vi "Main_011.vi"() -> ()   [LabVIEW 2025]
uses:
  Utility/Universal Utility/TypeDefs_Utility/ENUM_8 Directions U-D-L-R.ctl
  9e3f57c0-2ef8-4495-8287-c6a42a5fb955.vi
  <vilib>/Utility/error.llb/Trim Whitespace.vi
  <vilib>/Utility/error.llb/Trim Whitespace One-Sided.vi
  Utility/Universal Utility/TypeDefs_Utility/Cluster_Row-Column.ctl
  Utility/Universal Utility/TypeDefs_Utility/ENUM_4 Directions U-D-L-R.ctl
panel:
  out "Array":i32[][](array[numeric])
  in  "Puzzle Input":u64=4
  in  "Puzzle Target":u64=70600674
  in  "Data":string
  out "MATCH":bool
  out "Answer":u64
  # "MAX Product in Grid"
  # "Number of same direction numbers\n(Up, Down, Left, Right  Diaganal)"
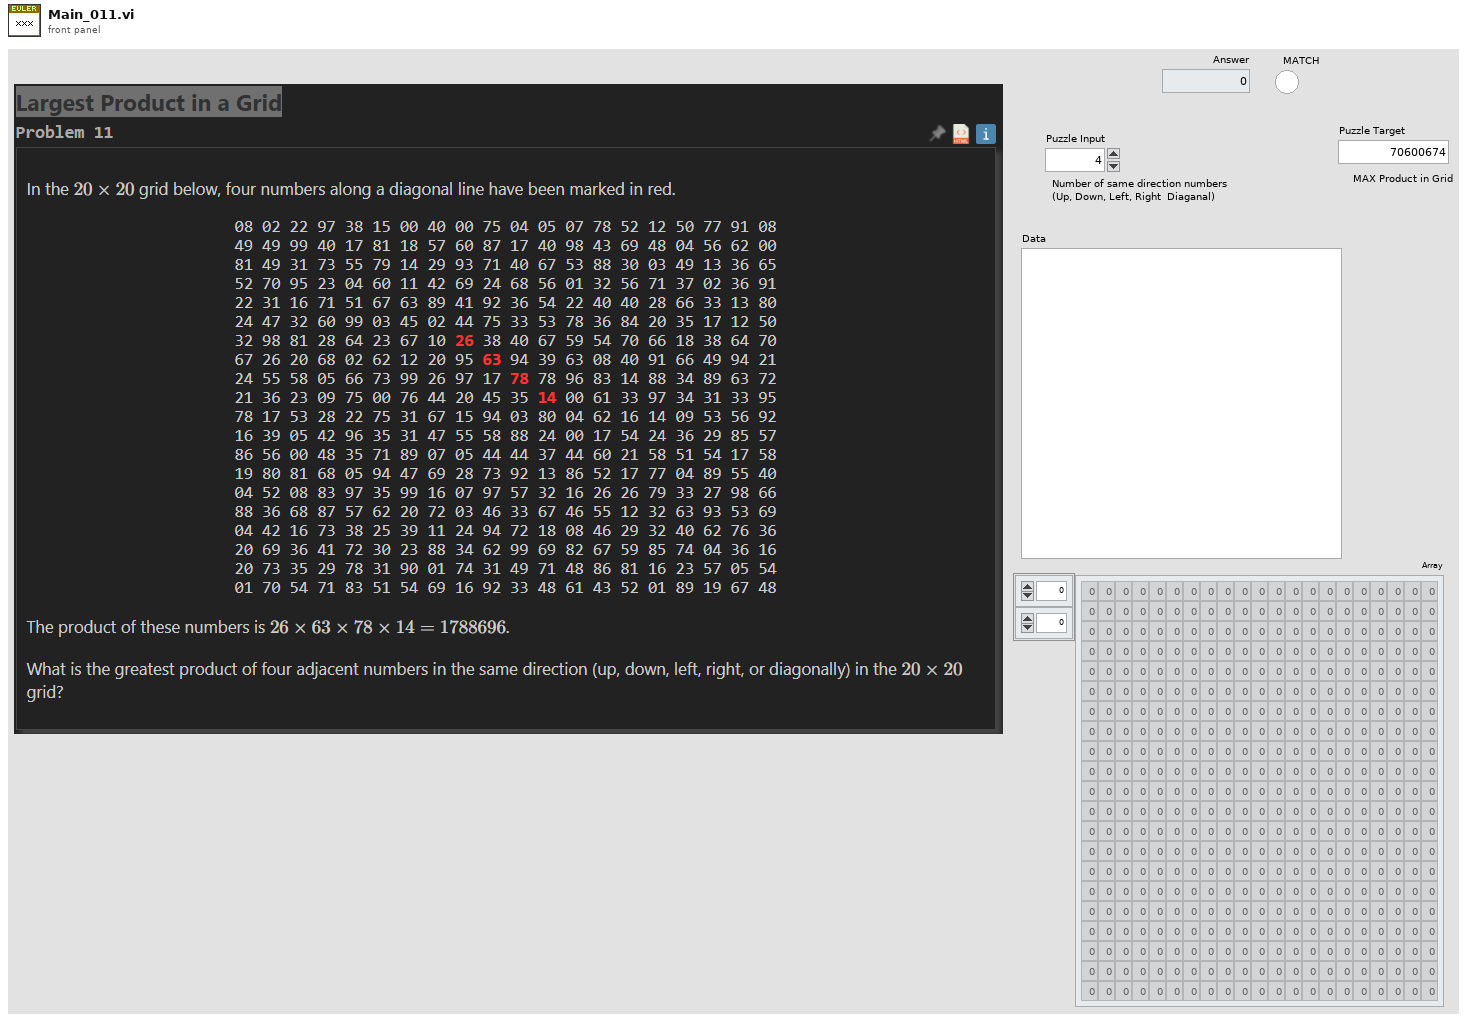
[diagram p1: front panel]
types:
  T1 = typedef "ENUM_4 Directions U-D-L-R.ctl" = enum16{"Up;-1,0", "Right;0,1", "Down;1,0", "Left;0,-1"}
  T2 = typedef "Cluster_Row-Column.ctl" = cluster{"R":i32, "C":i32}
  T3 = typedef "ENUM_8 Directions U-D-L-R.ctl" = enum16{"Up;-1,0", "Up-Right;-1,1", "Right;0,1", "Down-Right;1,1", "Down;1,0", "Down-Left;1,-1", "Left;0,-1", "Up-Left;-1,-1"}
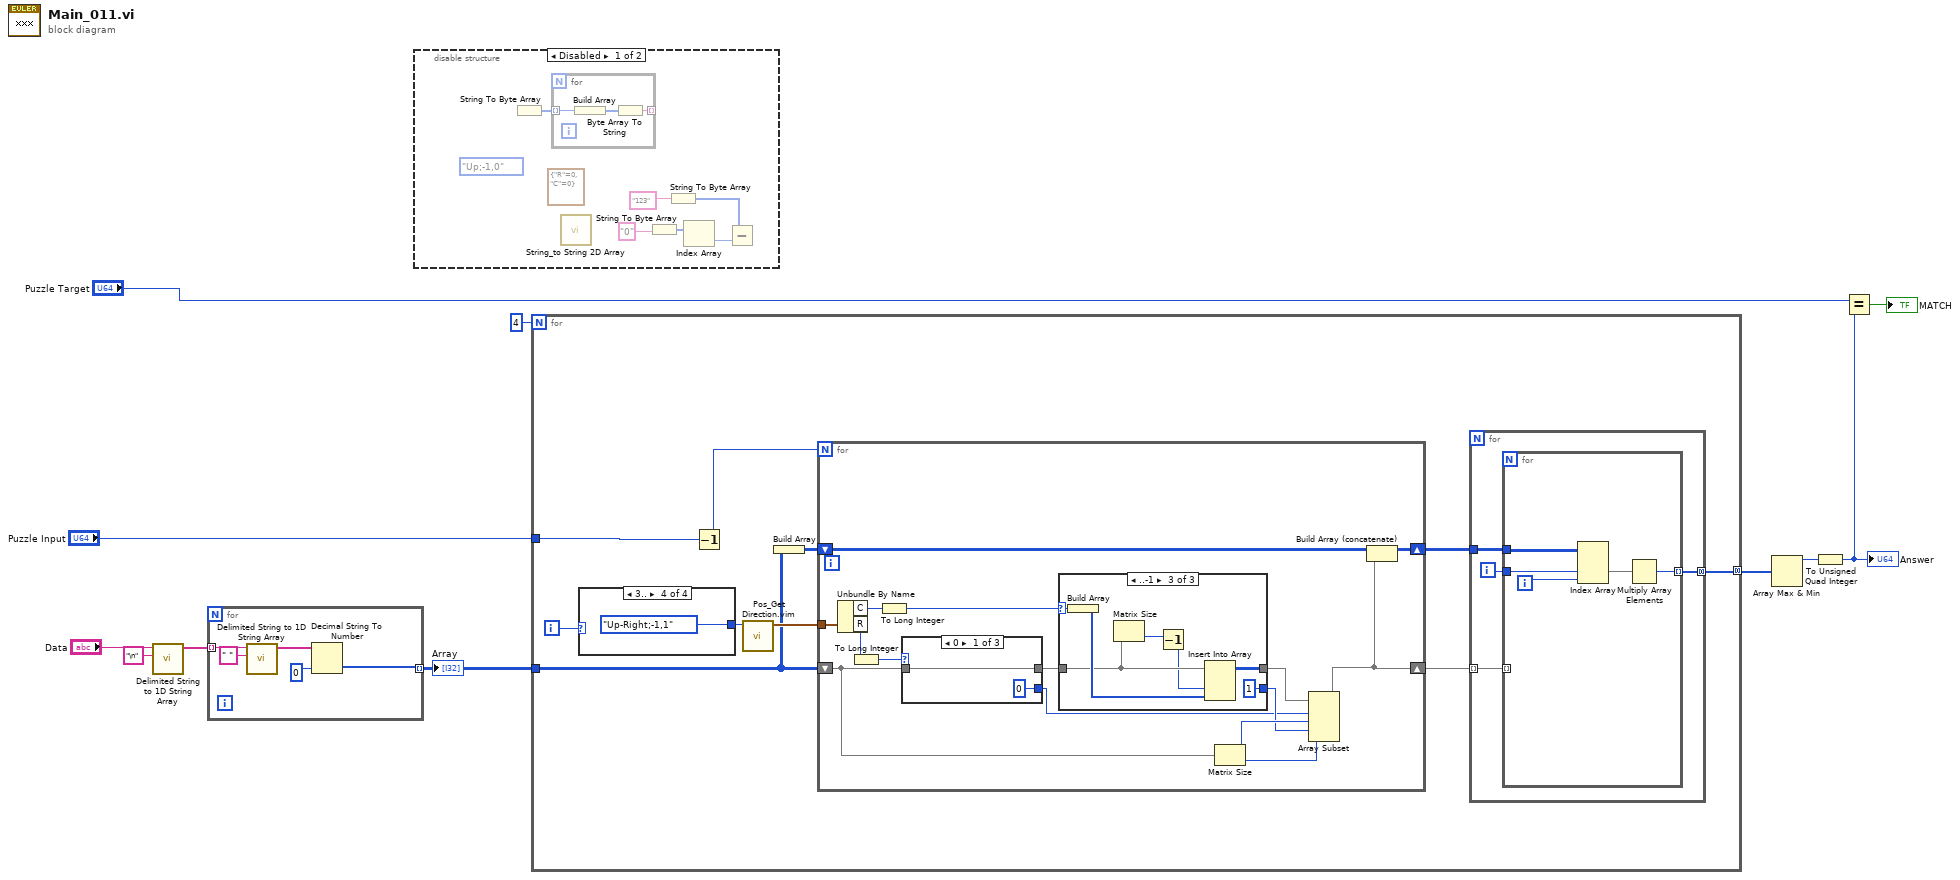
[diagram p0: block diagram]
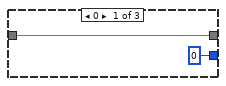
[diagram p2: hidden frame]
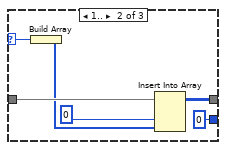
[diagram p3: hidden frame]
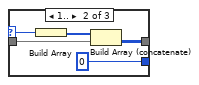
[diagram p4: hidden frame]
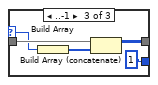
[diagram p5: hidden frame]
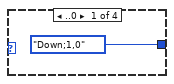
[diagram p6: hidden frame]
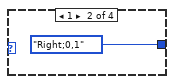
[diagram p7: hidden frame]
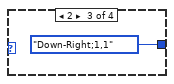
[diagram p8: hidden frame]
diagram:
  n1 = call <vilib>:"Delimited String to 1D String Array.vi"("delimiter"="\n", "delimited string"="Data") -> ("string array"=w6:string[])  [unwired: 9 in]
  n2 = for {
    tunnel: w6 -> [w16] mode=indexing
    tunnel: [w12] -> w4 mode=indexing
    n3 = call <vilib>:"Delimited String to 1D String Array.vi"("delimiter"=" ", "delimited string"=w16) -> ("string array"=w13:string[])  [unwired: 9 in]
    n4 = Decimal String To Number(string=w13, default (0L)=0 ("default (0 I32)")) -> (number=w12:i32[])  [unwired: 1 in, 1 out]
  }
  "Array" <- w4
  n5 = disable-structure shown="Disabled" {
    frame Disabled {
      (unwired) ENUM_4_Directions_U-D-L-R."Up;-1,0" ("Direction")
      (unwired) T2 {"R"=0, "C"=0} ("Position")
      n6 = String To Byte Array() -> (unsigned byte array=w17:u8[])  [unwired: 1 in]
      n7 = for {
        tunnel: w17 -> [w25] mode=indexing
        tunnel: [w23] -> _ mode=indexing
        n8 = Build Array(w25) -> (w24:u8[])
        n9 = Byte Array To String(unsigned byte array=w24) -> (string=w23:string)
      }
      n10 = call "String_to String 2D Array.vi"() -> ()  [unwired: 11 in, 1 out]
      n11 = String To Byte Array(string="0") -> (unsigned byte array=w20:u8[])
      n12 = String To Byte Array(string="123") -> (unsigned byte array=w18:u8[])
      n13 = Index Array(array=w20) -> (element=w19:u8)  [unwired: 1 in]
      n14 = Subtract(x=w18, y=w19) -> ()  [unwired: 1 out]
    }
    frame Enabled {
    }
  }
  n15 = for {
    N: 4 -> [_]
    tunnel: w4 -> [w32]
    tunnel: "Puzzle Input" -> [w30]
    tunnel: [w26] -> w2 mode=concatenating
    i -> [w35]
    n16 = case shown="3.." w35 {
      tunnel: [ENUM_8_Directions_U-D-L-R."Down;1,0" ("Direction 8") ENUM_8_Directions_U-D-L-R."Right;0,1" ("Direction 8") ENUM_8_Directions_U-D-L-R."Down-Right;1,1" ("Direction 8") ENUM_8_Directions_U-D-L-R."Up-Right;-1,1" ("Direction 8")] -> w34
      frame ..0 {
      }
      frame 1 {
      }
      frame 2 {
      }
      frame 3.. {
      }
    }
    n17 = Decrement(x=w30) -> (x-1=w29:u64)
    n18 = call "Pos_Get Direction.vim"("Direction 8"=w34) -> ("Position"=w33:T2)  [unwired: 10 in]
    n19 = Build Array(w32) -> (w31:i32[][][])
    n20 = for {
      N: w29 -> [_]
      tunnel: w33 -> [w59]
      shift-right: [w48] -> w28
      shift-left: w32 -> [w53]
      shift-right: [w49] -> w27
      shift-left: w31 -> [w50]
      n21 = Unbundle By Name(w59) -> ("C"=w56:i32, "R"=w58:i32)
      n22 = To Long Integer(number=w58) -> (32bit integer=w57:i32)
      n23 = To Long Integer(number=w56) -> (32bit integer=w55:i32)
      n24 = case shown="0" w57 {
        selector: w57 -> [_ w80 w85]
        tunnel: w53 -> [w76 w81 w86]
        tunnel: [w76 w78 w84] -> w54
        tunnel: [0 0 1] -> w45
        frame 0 {
        }
        frame 1.. {
          n25 = Build Array(w80) -> (w79:i32[])
          n26 = Build Array (concatenate)(w79, w81) -> (w78:i32[][])
        }
        frame ..-1 {
          n27 = Build Array(w85) -> (w82:i32[])
          n28 = Build Array (concatenate)(w86, w82) -> (w84:i32[][])
        }
      }
      n29 = case shown="..-1" w55 {
        selector: w55 -> [_ w67 w74]
        tunnel: w54 -> [w61 w66 w70]
        tunnel: [w61 w65 w73] -> w52
        tunnel: [0 0 1] -> w46
        frame 0 {
        }
        frame 1.. {
          n30 = Build Array(w67) -> (w63:i32[])
          n31 = Insert Into Array(array=w66, index (col)=0, new element=w63) -> (w65:i32[][])  [unwired: 1 in]
        }
        frame ..-1 {
          n32 = Build Array(w74) -> (w72:i32[])
          n33 = Matrix Size(0:w70) -> (2:w69:i32)  [unwired: 1 out]
          n34 = Decrement(x=w69) -> (x-1=w68:i32)
          n35 = Insert Into Array(array=w70, index (col)=w68, new element=w72) -> (w73:i32[][])  [unwired: 1 in]
        }
      }
      n36 = Matrix Size(0:w53) -> (1:w47:i32, 2:w51:i32)
      n37 = Array Subset(array=w52, index (row)=w45, length (row)=w47, index (col)=w46, length (col)=w51) -> (w48:i32[][])
      n38 = Build Array (concatenate)(w50, w48) -> (w49:i32[][][])
    }
    n39 = for {
      tunnel: w28 -> [w39] mode=indexing
      tunnel: w27 -> [w38]
      tunnel: [w36] -> w26 mode=concatenating
      i -> [w37]
      n40 = for {
        tunnel: w39 -> [_] mode=indexing
        tunnel: w38 -> [w44]
        tunnel: w37 -> [w43]
        tunnel: [w40] -> w36 mode=indexing
        i -> [w42]
        n41 = Index Array(array=w44, index (dim 1)=w43, index (dim 2)=w42) -> (element=w41:i32[])  [unwired: 1 in]
        n42 = Multiply Array Elements(1:w41) -> (0:w40:i32)
      }
    }
  }
  n43 = Array Max & Min(array=w2) -> (max value=w1:i32)  [unwired: 3 out]
  n44 = To Unsigned Quad Integer(1:w1) -> (0:w9:u64)
  "Answer" <- w9
  n45 = Equal?(x="Puzzle Target", y=w9) -> (x = y?=→"MATCH":bool)
